vi "Set Output State.vi"(8 "error in (no error)":errorcluster, 10 "Speed & Direction":i16, 11 "Reference Range Actor in":refnum<class "Reference Range Actor.lvclass">) -> (0 "error out":errorcluster, 3 "Reference Range Actor out":refnum<class "Reference Range Actor.lvclass">)   [LabVIEW 2018, in "Reference Range.lvlib" / "Reference Range Actor.lvclass"]
doc: "When setting the output state, the default value is '128' (Stop). Otherwise, '0' is full reverse and '255' is full forward, with incremental speeds in between."
uses:
  Reference Range Actor.lvclass
  C:/Program Files (x86)/National Instruments/LabVIEW 2018/vi.lib/ActorFramework/Actor/Actor.lvclass
  Reference Range Actor.lvclass/Reference Range Actor.ctl
  <vilib>/ActorFramework/Actor/Actor.lvclass/Actor.ctl
  <vilib>/ActorFramework/Actor/Actor.lvclass
  Range Controller Actor Messages/Send Log Message to Caller Msg/Send Log Message to Caller Msg.lvclass
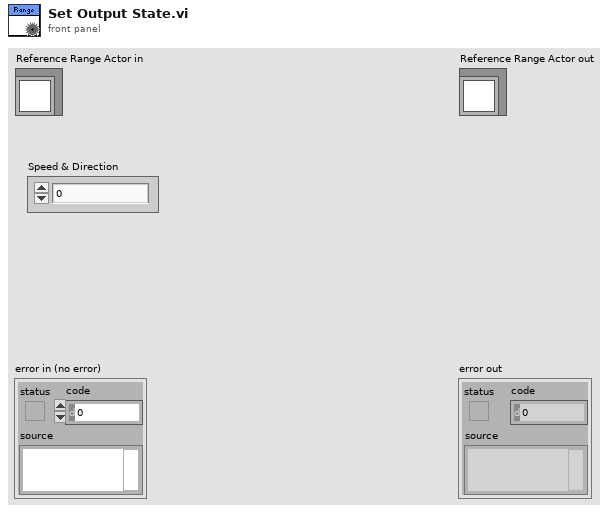
[diagram p1: front panel]
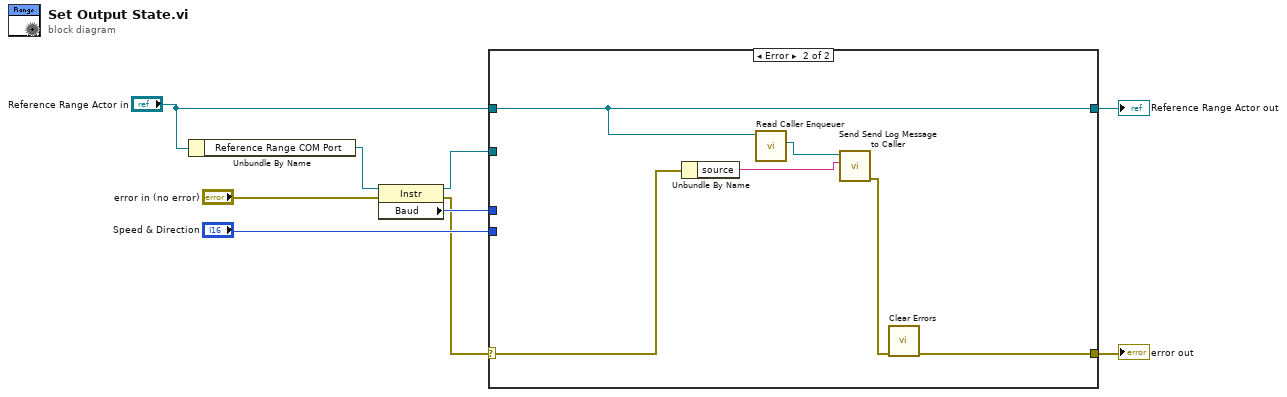
[diagram p0: block diagram]
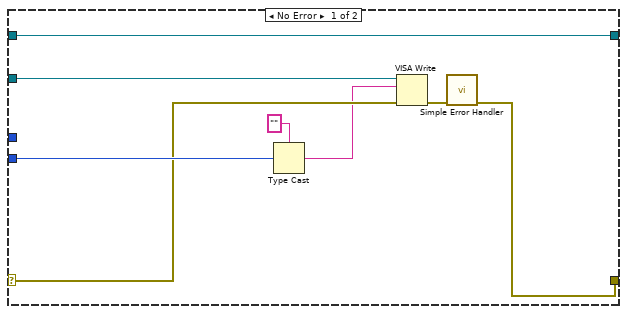
[diagram p2: hidden frame]
diagram:
  n1 = Unbundle By Name("Reference Range Actor in") -> ("Reference Range COM Port"=w5:refnum<visa-resource-name>)
  n2 = property class="Instr"(reference=w5, error in="error in (no error)") -> (reference out=w1:refnum<visa-resource-name>, error out=w2:errorcluster, "Baud"=w4:u32)
  n3 = case shown="Error" w2 {
    selector: w2 -> [w15 w19]
    tunnel: [w14 w23] -> w9
    tunnel: [w16 w22] -> w8
    tunnel: "Reference Range Actor in" -> [w16 w22]
    tunnel: "Speed & Direction" -> [w17 _]
    tunnel: w1 -> [w13 _]
    tunnel: w4 -> [_ _]
    frame No Error {
      n4 = Type Cast(type="", x=w17) -> (*(type *) &x=w11:string)
      n5 = VISA Write(VISA resource name=w13, write buffer=w11, error in (no error)=w15) -> (error out=w10:errorcluster)  [unwired: 2 out]
      n6 = call <vilib>:"Simple Error Handler.vi"("error in (no error)"=w10) -> ("error out"=w14:errorcluster)  [unwired: 4 in, 4 out]
    }
    frame Error {
      n7 = Unbundle By Name(w19) -> ("source"=w20:string)
      n8 = call <vilib>:"Read Caller Enqueuer.vi"("Actor"=w22) -> ("Caller Enqueuer"=w21:refnum<class "Message Enqueuer.lvclass">)  [unwired: 10 in]
      n9 = call "Send Send Log Message to Caller.vi"("Log Message"=w20, "Message Enqueuer in"=w21) -> ("error out"=w18:errorcluster)  [unwired: 8 in, 1 out]
      n10 = call <vilib>:"Clear Errors.vi"("error in (no error)"=w18) -> ("error out"=w23:errorcluster)  [unwired: 5 in, 1 out]
    }
  }
  "error out" <- w9
  "Reference Range Actor out" <- w8
